vi "4 DDS.vi"(9 "pdw in":T2 {"frequency shift" format="%#_12f"}, 10 "free DDS before me?":bool, 11 "new PDW in":bool) -> (1 "state of every DDS":bool[](array[boolean]), 2 "have free DDS":bool, 3 "IQ out":T1)   [LabVIEW 2021]
doc: "transmit pulse with one free DDS inside.\nmust have no DDS before him (the distribute is to give the lowest mun DDS the pulse)"
uses:
  pdw.ctl
  mode_type.ctl
  <instrlib>/_niInstr/DSP/v1/Shared/Public/IQ Data.ctl
  <instrlib>/_niInstr/DSP/v1/Shared/niInstr DSP v1 Shared.lvlib
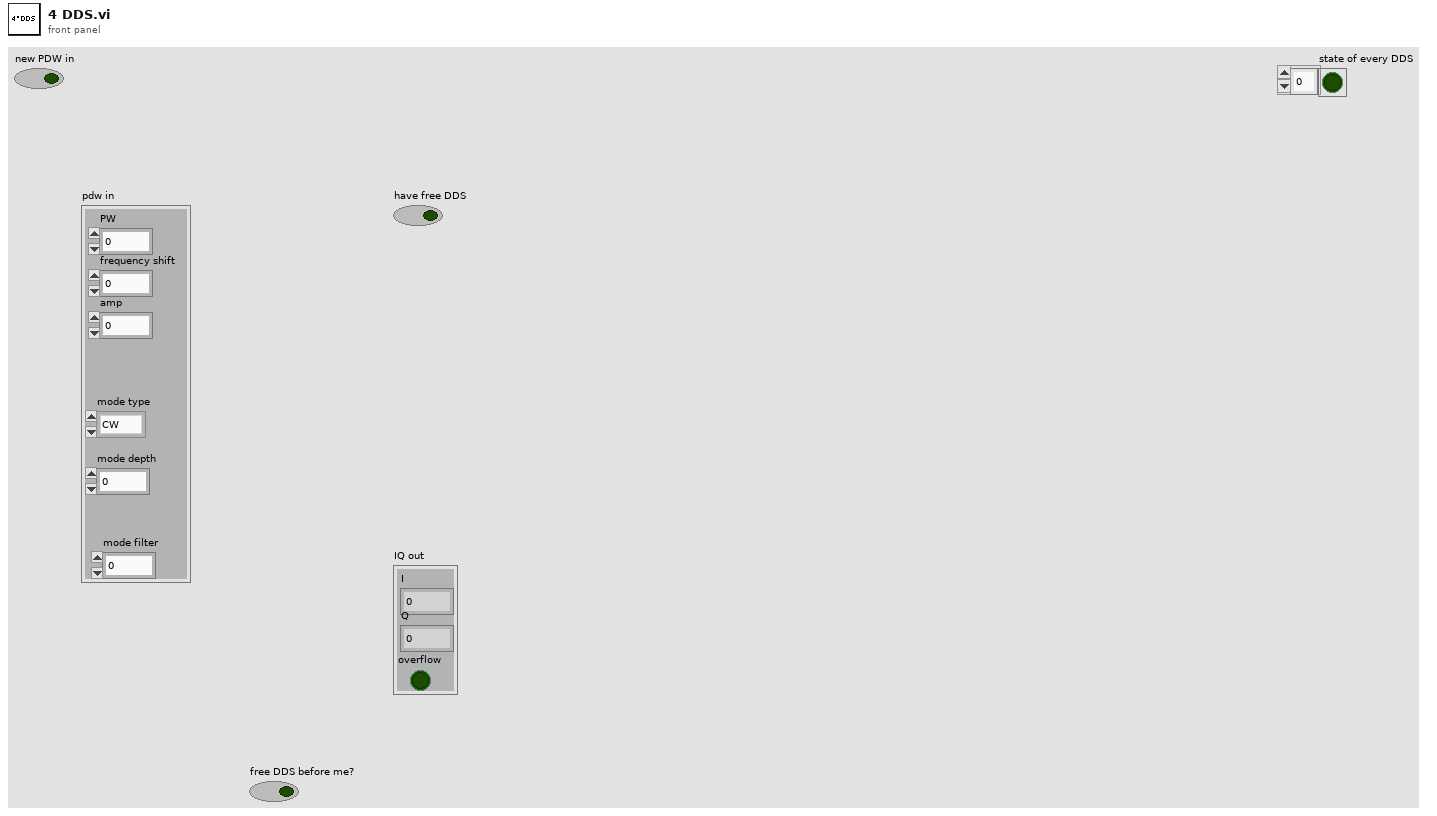
[diagram p1: front panel]
types:
  T1 = typedef "niInstr DSP v1 Shared.lvlib/IQ Data.ctl" = cluster{"I":fxp<+/-,18,1>, "Q":fxp<+/-,18,1>, "overflow":bool}
  T2 = typedef "pdw.ctl" = cluster{"PW":u32, "frequency shift":fxp<+/-,48,0>, "amp":fxp<+/-,18,1>, "mode type":T3, "mode depth":u32, "mode filter":u8}
  T3 = typedef "mode_type.ctl" = enum8{"CW", "NC - CW", "NC - cw", "LFM", "BPSK", "QPSK"}
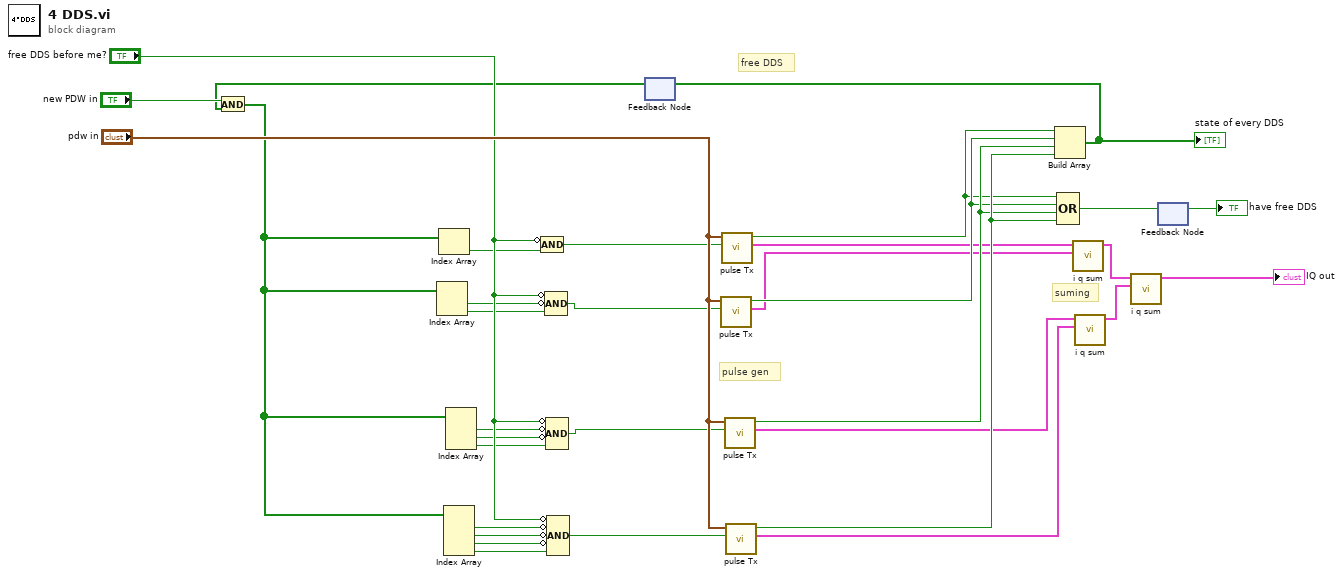
[diagram p0: block diagram]
diagram:
  # "free DDS"
  # "suming"
  # "pulse gen"
  n1 = feedback #1() -> (w4:bool[])  [unwired: 1 in]
  n2 = And(x="new PDW in", y=w4) -> (x .and. y?=w3:bool[])
  n3 = Index Array(array=w3) -> (element #1=w17:bool, element #2=w15:bool)  [unwired: 2 in]
  n4 = Index Array(array=w3) -> (element=w13:bool)  [unwired: 1 in]
  n5 = Index Array(array=w3) -> (element #1=w25:bool, element #2=w24:bool, element #3=w23:bool, element #4=w22:bool)  [unwired: 4 in]
  n6 = Index Array(array=w3) -> (element #1=w21:bool, element #2=w20:bool, element #3=w19:bool)  [unwired: 3 in]
  n7 = Compound Arithmetic op=AND(invert "free DDS before me?", w13) -> (w14:bool)
  n8 = Compound Arithmetic op=AND(invert "free DDS before me?", invert w17, w15) -> (w16:bool)
  n9 = Compound Arithmetic op=AND(invert "free DDS before me?", invert w21, invert w20, w19) -> (w18:bool)
  n10 = Compound Arithmetic op=AND(invert "free DDS before me?", invert w25, invert w24, invert w23, w22) -> (w26:bool)
  n11 = call "pulse Tx.vi"("take it!"=w16, "Cluster"="pdw in") -> ("data out"=w10:T1, "free dds"=w29:bool)  [unwired: 6 in, 2 out]
  n12 = call "pulse Tx.vi"("take it!"=w14, "Cluster"="pdw in") -> ("data out"=w9:T1, "free dds"=w28:bool)  [unwired: 6 in, 2 out]
  n13 = call "pulse Tx.vi"("take it!"=w18, "Cluster"="pdw in") -> ("data out"=w11:T1, "free dds"=w30:bool)  [unwired: 6 in, 2 out]
  n14 = call "pulse Tx.vi"("take it!"=w26, "Cluster"="pdw in") -> ("data out"=w12:T1, "free dds"=w31:bool)  [unwired: 6 in, 2 out]
  n15 = Build Array(w28, w29, w30, w31) -> (w6:bool[])
  "state of every DDS" <- w6
  n16 = feedback-in #1(w6) -> ()
  n17 = Compound Arithmetic op=OR(w28, w29, w30, w31) -> (w2:bool)
  n18 = call "i q sum.vi"(10:"data in"=w10, 11:"data in"=w9) -> ("output cluster"=w8:T1)  [unwired: 9 in]
  n19 = call "i q sum.vi"(10:"data in"=w12, 11:"data in"=w11) -> ("output cluster"=w7:T1)  [unwired: 9 in]
  n20 = call "i q sum.vi"(10:"data in"=w7, 11:"data in"=w8) -> ("output cluster"=→"IQ out":T1)  [unwired: 9 in]
  n21 = feedback #2() -> (→"have free DDS":bool)  [unwired: 1 in]
  n22 = feedback-in #2(w2) -> ()
